vi "Main.vi"(11 "Module Admin":refnum<class "Delacor_lib_QMH_Module Admin.lvclass">) -> ()   [LabVIEW 2025, in "Settings Editor.lvlib"]
doc: "This template is based off of the Queued Message Handler design pattern and the Queued Message Handler project template that ships with LabVIEW.\n\nThe main difference is that the queue is private to this module and communication between modules is performed via Broadcast and Request events.\n\nRequest events are wrapped in public API methods and are handled in the Event Handling Loop (EHL) of this VI. Any module can register for Broadcast events sent by this module. The EHL generates messages based on user interface actions.\n\nThe Message Handling Loop (MHL) processes messages generated by the EHL, or by other messages. The messages are string values, so new messages can be added easily to the Message Cases case structure in the MHL. Each message cluster can also provide an optional value for Message Data, which is a variant that can be converted to whatever message-specific data is required.\n_____\nBased on DQMH Project Template 4.0.0.47.\n_____\nBased on DQMH Dev Tools: Project Template 7.1.0.1503."
uses:
  Settings Editor.lvlib
  <vilib>/Delacor/Delacor QMH/Libraries/Module Admin_class/Delacor_lib_QMH_Module Admin.lvclass
  Test Meta Data.ctl
  Module Data--cluster.ctl
  Settings--cluster.ctl
  Stop Argument--cluster.ctl
  <vilib>/Delacor/Delacor QMH/Libraries/Message Queue_class/Delacor_lib_QMH_Message Queue.lvclass/Delacor_lib_QMH_Message Queue.ctl
  Update Application Settings Argument--cluster.ctl
  Update Application Settings (Reply Payload)--cluster.ctl
  <vilib>/Delacor/Delacor QMH/Libraries/Module Admin_class/Delacor_lib_QMH_Module Admin.lvclass/Delacor_lib_QMH_Module Admin.ctl
  Udate Test Meta Data Argument--cluster.ctl
  Save Test Meta Data (Reply Payload)--cluster.ctl
  <vilib>/Utility/miscctls.llb/LVPointTypeDef.ctl
  <vilib>/Delacor/Delacor QMH/Libraries/Message Queue_class/Delacor_lib_QMH_Enqueue Message (Single).vi
  <vilib>/Delacor/Delacor QMH/Libraries/Module Admin_class/Delacor_lib_QMH_Get External Launch.vi
  <vilib>/Delacor/Delacor QMH/Libraries/Message Queue_class/Delacor_lib_QMH_Message Queue.lvclass
panel:
  in  "Report Save Path":path
  in  "DAQ Settings":T1
  in  "Test Meta Data":T2
  in  "Cancel":bool
  in  "OK":bool
  in  "Log File Base Path":path
  out "error out":errorcluster
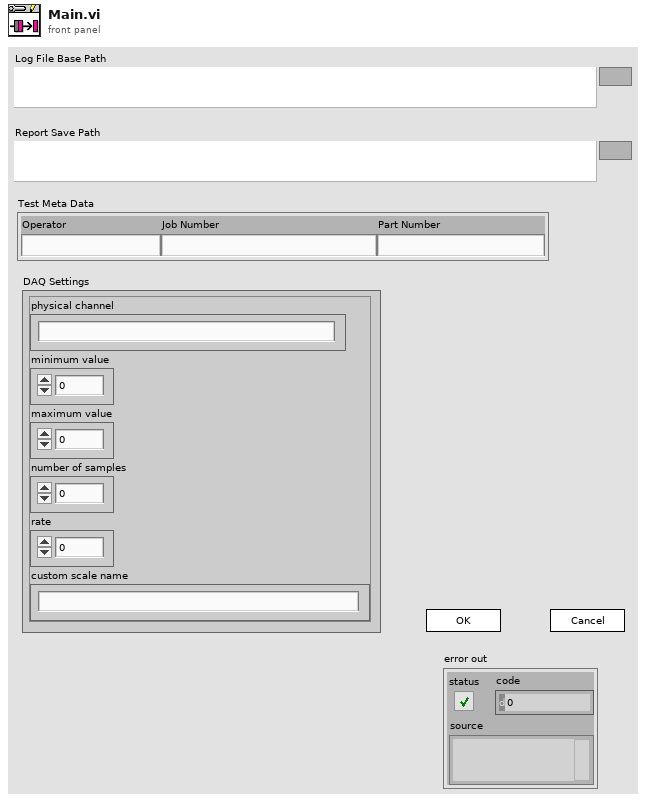
[diagram p1: front panel]
types:
  T1 = cluster{"physical channel":string, "minimum value":dbl, "maximum value":dbl, "number of samples":i32, "rate":dbl, "custom scale name":string}
  T2 = typedef "Settings Editor.lvlib/Test Meta Data.ctl" = cluster{"Operator":string, "Job Number":string, "Part Number":string}
  T3 = typedef "Settings Editor.lvlib/Request Events--cluster.ctl" = cluster{"Stop Module":refnum<user-event>, "Show Panel":refnum<user-event>, "Hide Panel":refnum<user-event>, "Get Module Execution Status":refnum<user-event>, "Show Diagram":refnum<user-event>, "Update Application Settings":refnum<user-event>, "Save Test Meta Data":refnum<user-event>}
  T4 = typedef "Settings Editor.lvlib/Module Data--cluster.ctl" = cluster{"Settings":T5}
  T5 = typedef "Settings Editor.lvlib/Settings--cluster.ctl" = cluster{"Log File Base Path":path, "Meta Data":T2, "DAQ Settings":cluster{"physical channel":string, "minimum value":dbl, "maximum value":dbl, "number of samples":i32, "rate":dbl, "custom scale name":string}, "Report Save Folder":path}
  T6 = enum32{"invalid lock state", "Not Locked", "Locked (No Password)", "Password-protected"}
  T7 = typedef "Settings Editor.lvlib/Stop Argument--cluster.ctl" = cluster{"Origin":string, "Exit via Stop Module Req?":bool, "Wait for Module to stop?":bool}
  T8 = typedef "Settings Editor.lvlib/Update Application Settings Argument--cluster.ctl" = cluster{"Wait Notifier":refnum<notifier>, "wait for reply":bool}
  T9 = typedef "Settings Editor.lvlib/Udate Test Meta Data Argument--cluster.ctl" = cluster{"Test Meta Data":T2, "Wait Notifier":refnum<notifier>, "wait for reply":bool}
  T10 = typedef "LVPointTypeDef.ctl" = cluster{"Horizontal":i16, "Vertical":i16}
  T11 = enum32{"Invalid", "Standard", "Closed", "Hidden", "Minimized", "Maximized"}
  T12 = typedef "Settings Editor.lvlib/Update Application Settings (Reply Payload)--cluster.ctl" = cluster{"Settings":T5, "error":errorcluster}
  T13 = typedef "Settings Editor.lvlib/Save Test Meta Data (Reply Payload)--cluster.ctl" = cluster{"error":errorcluster}
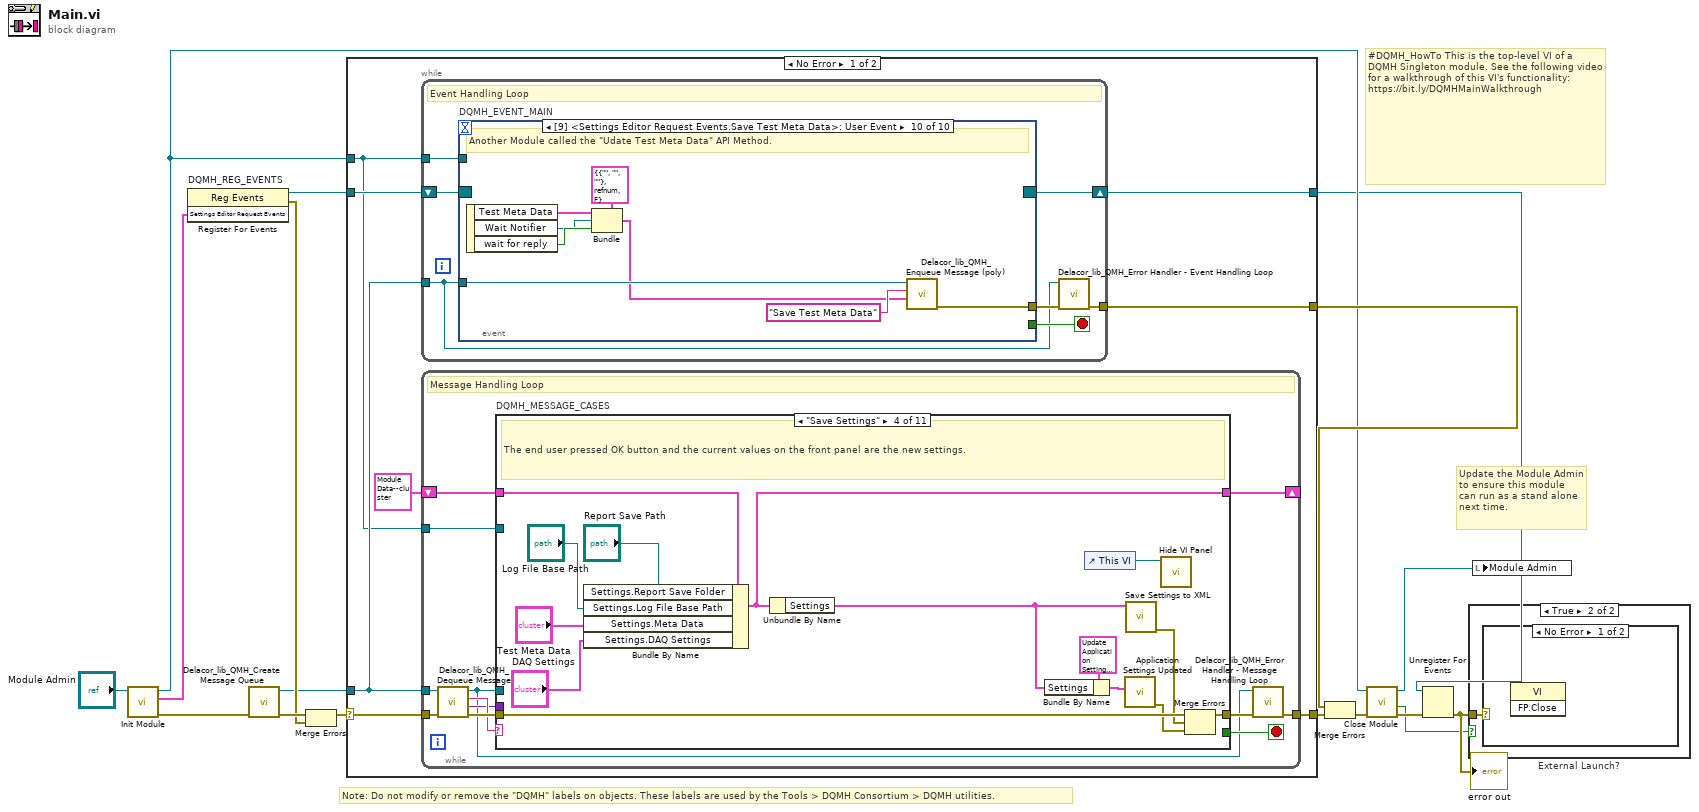
[diagram p0: block diagram]
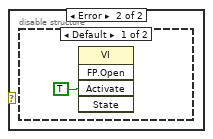
[diagram p3: hidden frame]
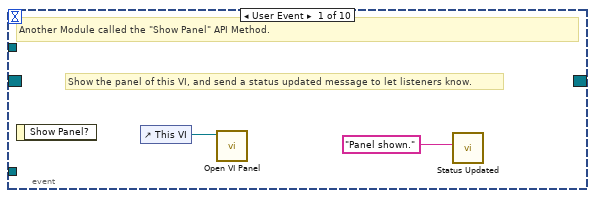
[diagram p5: hidden frame]
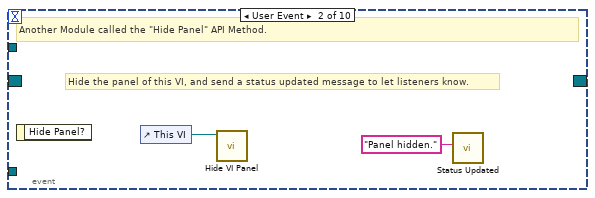
[diagram p6: hidden frame]
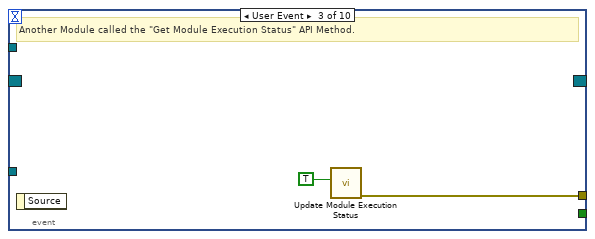
[diagram p7: hidden frame]
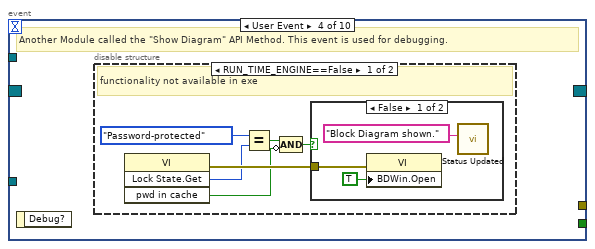
[diagram p8: hidden frame]
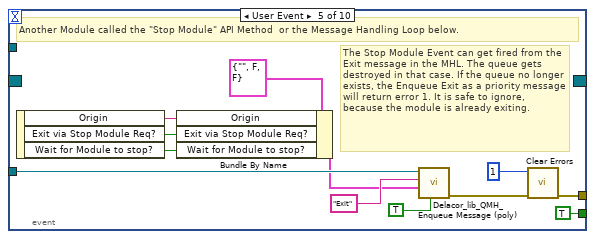
[diagram p11: hidden frame]
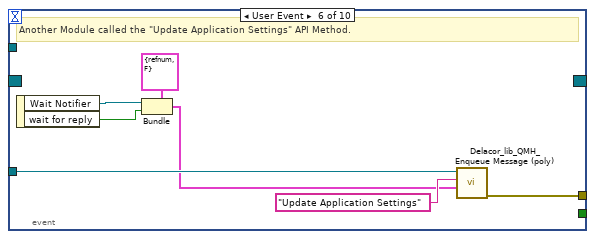
[diagram p12: hidden frame]
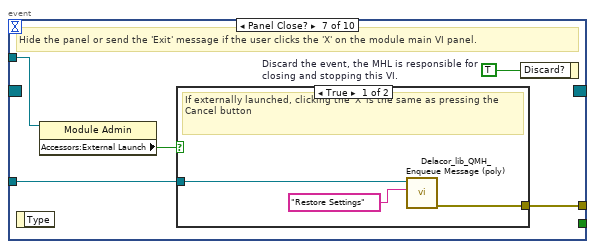
[diagram p13: hidden frame]
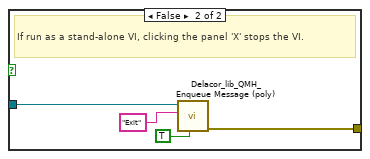
[diagram p14: hidden frame]
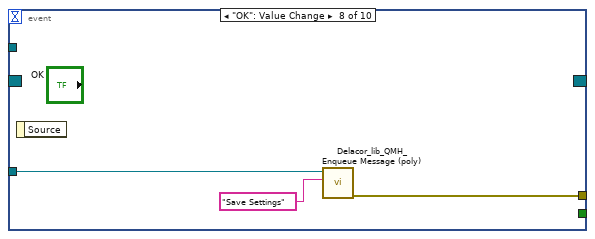
[diagram p15: hidden frame]
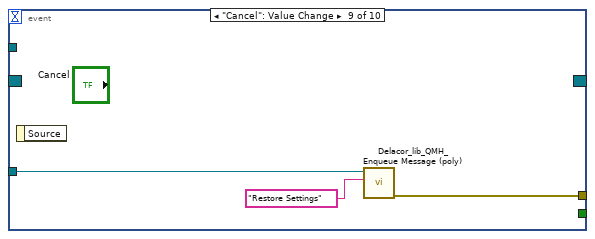
[diagram p16: hidden frame]
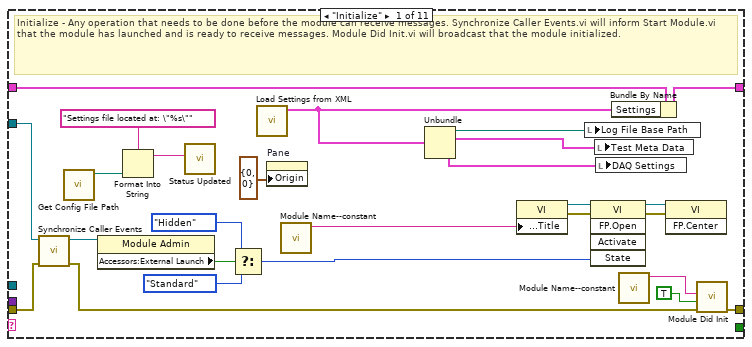
[diagram p17: hidden frame]
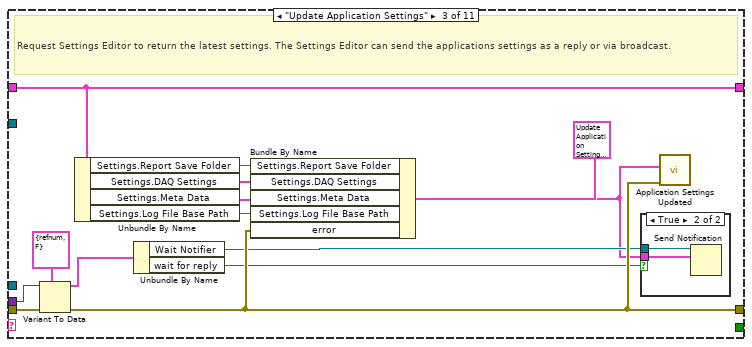
[diagram p19: hidden frame]
diagram:
  # "#DQMH_HowTo This is the top-level VI of a DQMH Singleton module. See the following video for a walkthrough of this VI's functionality: https://bit.ly/DQMHMainWalkthrough"
  # "Note: Do not modify or remove the \"DQMH\" labels on objects. These labels are used by the Tools > DQMH Consortium > DQMH utilities."
  # "Update the Module Admin to ensure this module can run as a stand alone next time."
  n1 = call "Init Module.vi"("Singleton Module Admin in"="Module Admin") -> ("error out"=w16:errorcluster, "Settings Editor Request Events"=w5:T3, "Singleton Module Admin out"=w8:refnum<class "Delacor_lib_QMH_Module Admin.lvclass">)  [unwired: 8 in]
  n2 = register-events "DQMH_REG_EVENTS"(w5) -> (reference out=w6:refnum<event-registration>, error out=w9:errorcluster)  [unwired: 2 in]
  n3 = call <vilib>:"Delacor_lib_QMH_Create Message Queue.vi"("error in"=w16) -> ("error out"=w11:errorcluster, "Message Queue"=w4:refnum<class "Delacor_lib_QMH_Message Queue.lvclass">)  [unwired: 9 in]
  n4 = Merge Errors(w11, w9) -> (w10:errorcluster)
  n5 = case shown="No Error" w10 {
    selector: w10 -> [w23 w244]
    tunnel: [w25 w243] -> w17
    tunnel: [w22 w242] -> w7
    tunnel: w6 -> [w20 w242]
    tunnel: w4 -> [w19 w237]
    tunnel: [w24 _] -> w14
    tunnel: w8 -> [w18 w238]
    frame No Error {
      n6 = while {
        tunnel: w19 -> [w26]
        shift-right: [w29] -> w22
        shift-left: w20 -> [w30]
        tunnel: [w31] -> w24
        tunnel: w18 -> [w27]
        stop <- w28 stop-if-true
        # "Event Handling Loop"
        n7 = event "DQMH_EVENT_MAIN" shown="[9] <Settings Editor Request Events.Save Test Meta Data>: User Event" {
          selector: w30 -> [_ _ _ _ _ _ _ _ _ _]
          dyn-events: [_ _ _ _ _ _ _ _ _ _] -> w29
          timeout: _ -> [_ _ _ _ _ _ _ _ _ _]
          tunnel: [_ _ _ _ TRUE ("Discard?") _ _ _ _ _] -> w28
          tunnel: w26 -> [_ _ _ _ w55 w65 w69 w79 w82 w92]
          tunnel: [_ _ w38 _ w58 w66 w71 w81 w84 w87] -> w32
          tunnel: w27 -> [_ _ _ _ _ _ w68 _ _ _]
          event User Event {
            # "Show the panel of this VI, and send a status updated message to let listeners know."
            # "Another Module called the \"Show Panel\" API Method."
            n8 = event-data() -> ()  [unwired: 1 in, 1 out]
            n9 = control-ref of="This VI"() -> (w34:refnum<vi>)
            n10 = call "Open VI Panel.vi"("VI"=w34) -> ()  [unwired: 10 in, 1 out]
            n11 = call "Status Updated.vi"("Status"="Panel shown." ("format string")) -> ()  [unwired: 10 in, 1 out]
          }
          event User Event {
            # "Hide the panel of this VI, and send a status updated message to let listeners know."
            # "Another Module called the \"Hide Panel\" API Method."
            n12 = event-data() -> ()  [unwired: 1 in, 1 out]
            n13 = control-ref of="This VI"() -> (w36:refnum<vi>)
            n14 = call "Hide VI Panel.vi"("VI"=w36) -> ()  [unwired: 10 in, 1 out]
            n15 = call "Status Updated.vi"("Status"="Panel hidden." ("format string")) -> ()  [unwired: 10 in, 1 out]
          }
          event User Event {
            # "Another Module called the \"Get Module Execution Status\" API Method."
            n16 = event-data() -> ()  [unwired: 1 in, 1 out]
            n17 = call "Update Module Execution Status.vi"("Running?"=TRUE) -> ("error out"=w38:errorcluster)  [unwired: 10 in]
          }
          event User Event {
            # "Another Module called the \"Show Diagram\" API Method. This event is used for debugging."
            n18 = event-data() -> ()  [unwired: 1 in, 1 out]
            n19 = disable-structure shown="RUN_TIME_ENGINE==False" {
              frame condition #0 (active) {
                # "functionality not available in exe"
                n20 = invoke on="Invoke Node" class="VI" method="Lock State.Get"() -> (error out=w44:errorcluster, "Get Lock State"=w43:T6, "pwd in cache"=w40:bool)  [unwired: 4 in, 1 out]
                n21 = Equal?(x=T6."Password-protected", y=w43) -> (x = y?=w41:bool)
                n22 = Compound Arithmetic op=AND(w41, invert w40) -> (w39:bool)
                n23 = case shown="False" w39 {
                  tunnel: w44 -> [w47 _]
                  frame False {
                    n24 = property on="Property Node" class="VI"(error in=w47, "BDWin.Open"=TRUE ("Block Diagram Window:Open")) -> ()  [unwired: 1 in, 2 out]
                    n25 = call "Status Updated.vi"("Status"="Block Diagram shown." ("format string")) -> ()  [unwired: 10 in, 1 out]
                  }
                  frame True {
                    # "Password-protected VI, and the password is not in the cache. Do not show the diagram."
                  }
                }
              }
              frame condition #1 {
              }
            }
          }
          event User Event {
            # "The Stop Module Event can get fired from the Exit message in the MHL. The queue gets destroyed in that case. If the queue no longer exists, the Enqueue Exit as a priority message will return error 1. It is safe to ignore, because the module is already exiting."
            # "Another Module called the \"Stop Module\" API Method  or the Message Handling Loop below."
            n26 = event-data() -> ("Origin"=w48:string, "Exit via Stop Module Req?"=w51:bool, "Wait for Module to stop?"=w50:bool)  [unwired: 1 in]
            n27 = Bundle By Name(cluster=T7 {"Origin"="", "Exit via Stop Module Req?"=FALSE, "Wait for Module to stop?"=FALSE} ("Stop Argument"), "Origin"=w48, "Exit via Stop Module Req?"=w51, "Wait for Module to stop?"=w50) -> (w49:T7)
            n28 = call-poly <vilib>:"Delacor_lib_QMH_Enqueue Message (poly).vi"("Priority Message? (F)"=TRUE, "Message Data"=w49, "Message"="Exit", "Message Queue in"=w55) -> ("error out"=w59:errorcluster)  [unwired: 6 in, 1 out]
            n29 = call <vilib>:"Clear Errors.vi"("error in (no error)"=w59, "specific error code to clear (0: all)"=1) -> ("error out"=w58:errorcluster)  [unwired: 4 in, 1 out]
          }
          event User Event {
            # "Another Module called the \"Update Application Settings\" API Method."
            n30 = event-data() -> ("Wait Notifier"=w61:refnum<notifier>, "wait for reply"=w60:bool)  [unwired: 1 in]
            n31 = Bundle(cluster=T8 {"Wait Notifier"=refnum, "wait for reply"=FALSE} ("Update Application Settings Argument"), "Wait Notifier"=w61, "wait for reply"=w60) -> (w62:T8)
            n32 = call-poly <vilib>:"Delacor_lib_QMH_Enqueue Message (poly).vi"("Message Data"=w62, "Message"="Update Application Settings", "Message Queue in"=w65) -> ("error out"=w66:errorcluster)  [unwired: 7 in, 1 out]
          }
          event Panel Close? {
            w70 = TRUE  # Discard the event, the MHL is responsible for closing and stopping this VI.
            # "Hide the panel or send the 'Exit' message if the user clicks the 'X' on the module main VI panel."
            n33 = event-data() -> ()  [unwired: 1 in, 1 out]
            n34 = property on="Property Node" class="Module Admin"(reference=w68) -> ("Accessors:External Launch"=w67:bool)  [unwired: 1 in, 2 out]
            n35 = case shown="True" w67 {
              tunnel: w69 -> [w72 w77]
              tunnel: [w74 w78] -> w71
              frame True {
                # "If externally launched, clicking the 'X' is the same as pressing the Cancel button"
                n36 = call-poly <vilib>:"Delacor_lib_QMH_Enqueue Message (poly).vi"("Message"="Restore Settings", "Message Queue in"=w72) -> ("error out"=w74:errorcluster)  [unwired: 8 in, 1 out]
              }
              frame False {
                # "If run as a stand-alone VI, clicking the panel 'X' stops the VI."
                n37 = call-poly <vilib>:"Delacor_lib_QMH_Enqueue Message (poly).vi"("Priority Message? (F)"=TRUE, "Message"="Exit", "Message Queue in"=w77) -> ("error out"=w78:errorcluster)  [unwired: 7 in, 1 out]
              }
            }
            n38 = event-data ("Event Filter Node")("Discard?"=w70) -> ()  [unwired: 1 in, 1 out]
          }
          event "OK": Value Change {
            n39 = event-data() -> ()  [unwired: 1 in, 1 out]
            n40 = call-poly <vilib>:"Delacor_lib_QMH_Enqueue Message (poly).vi"("Message"="Save Settings", "Message Queue in"=w79) -> ("error out"=w81:errorcluster)  [unwired: 8 in, 1 out]
          }
          event "Cancel": Value Change {
            n41 = event-data() -> ()  [unwired: 1 in, 1 out]
            n42 = call-poly <vilib>:"Delacor_lib_QMH_Enqueue Message (poly).vi"("Message"="Restore Settings", "Message Queue in"=w82) -> ("error out"=w84:errorcluster)  [unwired: 8 in, 1 out]
          }
          event User Event {
            # "Another Module called the \"Udate Test Meta Data\" API Method."
            n43 = event-data() -> ("Test Meta Data"=w88:T2, "Wait Notifier"=w85:refnum<notifier>, "wait for reply"=w86:bool)  [unwired: 1 in]
            n44 = Bundle(cluster=T9 {"Test Meta Data"={"Operator"="", "Job Number"="", "Part Number"=""}, "Wait Notifier"=refnum, "wait for reply"=FALSE} ("Udate Test Meta Data Argument"), "Test Meta Data"=w88, "Wait Notifier"=w85, "wait for reply"=w86) -> (w89:T9)
            n45 = call-poly <vilib>:"Delacor_lib_QMH_Enqueue Message (poly).vi"("Message Data"=w89, "Message"="Save Test Meta Data", "Message Queue in"=w92) -> ("error out"=w87:errorcluster)  [unwired: 7 in, 1 out]
          }
        }
        n46 = call-dynamic "Delacor_lib_QMH_Error Handler - Event Handling Loop.vi"("error in"=w32, "Message Queue in"=w26) -> ("dup error in"=w31:errorcluster)  [unwired: 8 in, 1 out]
      }
      n47 = while {
        tunnel: w19 -> [w95]
        shift-right: [w99] -> _
        shift-left: T4 {"Settings"={"Log File Base Path"=path "", "Meta Data"={"Operator"="", "Job Number"="", "Part Number"=""}, "DAQ Settings"={"physical channel"="cDAQ9181-1913300Mod1/ai0", "minimum value"=0.0, "maximum value"=94400.0, "number of samples"=10, "rate"=125.0, "custom scale name"="Pressure"}, "Report Save Folder"=path ""}} ("Data Cluster") -> [w100]
        tunnel: w23 -> [w103]
        tunnel: [w101] -> w25
        tunnel: w18 -> [w93]
        stop <- w98 stop-if-true
        # "Message Handling Loop"
        n48 = call-dynamic "Delacor_lib_QMH_Dequeue Message.vi"("error in"=w103, "Message Queue in"=w95) -> ("error out"=w102:errorcluster, "Message Data"=w96:variant, "Message"=w97:string, "Message Queue out"=w94:refnum<class "Delacor_lib_QMH_Message Queue.lvclass">)  [unwired: 6 in]
        n49 = case "DQMH_MESSAGE_CASES" shown="\"Save Settings\"" w97 {
          selector: w97 -> [_ _ _ _ _ _ _ _ _ _ w232]
          tunnel: w94 -> [_ _ _ _ _ _ _ _ w198 w220 _]
          tunnel: w102 -> [w129 w132 w145 w161 w170 w187 w192 w194 w205 w226 w235]
          tunnel: [w127 w132 w146 w162 w170 w178 w191 w194 w201 w221 w236] -> w104
          tunnel: w100 -> [w117 w131 w139 w158 w169 w174 w190 w193 w200 w219 w233]
          tunnel: [w116 w131 w139 w156 w169 w172 w190 w193 w200 w219 w233] -> w99
          tunnel: [_ _ _ _ _ _ _ _ _ w218 _] -> w98
          tunnel: w96 -> [_ _ w144 _ _ w185 _ _ w199 w217 _]
          tunnel: w93 -> [w118 _ _ _ _ _ _ _ w197 w212 _]
          frame "Initialize" {
            # "Initialize - Any operation that needs to be done before the module can receive messages. Synchronize Caller Events.vi will inform Start Module.vi that the module has launched and is ready to receive messages. Module Did Init.vi will broadcast that the module initialized."
            n50 = call "Synchronize Caller Events.vi"("error in"=w129, "Singleton Module Admin in"=w118) -> ("error out"=w128:errorcluster, "Singleton Module Admin out"=w113:refnum<class "Delacor_lib_QMH_Module Admin.lvclass">)  [unwired: 8 in]
            n51 = call "Get Config File Path.vi"() -> ("XML File Path"=w111:path)  [unwired: 10 in, 1 out]
            n52 = property on="Property Node" class="Module Admin"(reference=w113) -> ("Accessors:External Launch"=w122:bool)  [unwired: 1 in, 2 out]
            n53 = Format Into String(format string="Settings file located at: \"%s\"", w111) -> (resulting string=w110:string)  [unwired: 2 in, 1 out]
            n54 = call "Status Updated.vi"("Status"=w110) -> ()  [unwired: 10 in, 1 out]
            n55 = Select(t=T11."Hidden" ("State"), s=w122, f=T11."Standard" ("State")) -> (s? t:f=w119:T11)
            n56 = call "Load Settings from XML.vi"() -> ("Settings out"=w107:T5)  [unwired: 10 in, 1 out]
            n57 = property on="Pane" class="Pane"("Origin"=T10 {"Horizontal"=0, "Vertical"=0}) -> ()  [unwired: 2 in, 2 out]
            n58 = call "Module Name--constant.vi"() -> ("Module Name"=w125:string)  [unwired: 11 in]
            n59 = Unbundle(w107) -> ("Log File Base Path"=w108:path, "Meta Data"=w106:T2, "DAQ Settings"=w105:T1)  [unwired: 1 out]
            n60 = property on="Property Node" class="VI"("Front Panel.Title"=w125) -> (reference out=w124:refnum<vi>, error out=w126:errorcluster)  [unwired: 2 in]
            n61 = local write "Log File Base Path"(w108) -> ()
            n62 = invoke on="Invoke Node" class="VI" method="FP.Open"(reference=w124, error in=w126, "State"=w119) -> (reference out=w123:refnum<vi>, error out=w130:errorcluster)  [unwired: 2 in, 3 out]
            n63 = local write "Test Meta Data"(w106) -> ()
            n64 = local write "DAQ Settings"(w105) -> ()
            n65 = Bundle By Name(cluster=w117, "Settings"=w107) -> (w116:T4)
            n66 = call "Module Name--constant.vi"() -> ("Module Name"=w114:string)  [unwired: 11 in]
            n67 = invoke on="Invoke Node" class="VI" method="FP.Center"(reference=w123, error in=w130) -> ()  [unwired: 1 in, 3 out]
            n68 = call "Module Did Init.vi"("error in"=w128, "Initialized?"=TRUE, "Origin"=w114) -> ("error out"=w127:errorcluster)  [unwired: 8 in]
          }
          frame "---Module Specific---" {
            # "Separator -- The following cases handle messages specific to this Module."
          }
          frame "Update Application Settings" {
            # "Request Settings Editor to return the latest settings. The Settings Editor can send the applications settings as a reply or via broadcast."
            n69 = Variant To Data(error in=w145, type=T8 {"Wait Notifier"=refnum, "wait for reply"=FALSE} ("Update Application Settings Argument"), Variant=w144) -> (data=w142:T8, error out=w146:errorcluster)
            n70 = Unbundle By Name(w139) -> ("Settings.Report Save Folder"=w133:path, "Settings.DAQ Settings"=w134:T1, "Settings.Meta Data"=w135:T2, "Settings.Log File Base Path"=w137:path)
            n71 = Unbundle By Name(w142) -> ("Wait Notifier"=w141:refnum<notifier>, "wait for reply"=w140:bool)
            n72 = Bundle By Name(cluster=T12 {"Settings"={"Log File Base Path"=path "", "Meta Data"={"Operator"="", "Job Number"="", "Part Number"=""}, "DAQ Settings"={"physical channel"="cDAQ9181-1913300Mod1/ai0", "minimum value"=0.0, "maximum value"=94400.0, "number of samples"=10, "rate"=125.0, "custom scale name"="Pressure"}, "Report Save Folder"=path ""}, "error"={"status"=FALSE, "code"=0, "source"=""}} ("Update Application Settings (Reply Payload)"), "Settings.Report Save Folder"=w133, "Settings.DAQ Settings"=w134, "Settings.Meta Data"=w135, "Settings.Log File Base Path"=w137, "error"=w146) -> (w136:T12)
            n73 = case shown="True" w140 {
              tunnel: w141 -> [_ w148]
              tunnel: w136 -> [_ w147]
              frame False {
              }
              frame True {
                n74 = Send Notification(notification=w147, notifier=w148) -> ()  [unwired: 1 in, 2 out]
              }
            }
            n75 = call "Application Settings Updated.vi"("error in"=w146, "Reply Payload"=w136) -> ()  [unwired: 9 in, 1 out]
          }
          frame "Save Settings" {
            # "The end user pressed OK button and the current values on the front panel are the new settings."
            n76 = Bundle By Name(cluster=w158, "Settings.Report Save Folder"="Report Save Path", "Settings.Log File Base Path"="Log File Base Path", "Settings.Meta Data"="Test Meta Data", "Settings.DAQ Settings"="DAQ Settings") -> (w156:T4)
            n77 = Unbundle By Name(w156) -> ("Settings"=w152:T5)
            n78 = Bundle By Name(cluster=T12 {"Settings"={"Log File Base Path"=path "", "Meta Data"={"Operator"="", "Job Number"="", "Part Number"=""}, "DAQ Settings"={"physical channel"="cDAQ9181-1913300Mod1/ai0", "minimum value"=0.0, "maximum value"=94400.0, "number of samples"=10, "rate"=125.0, "custom scale name"="Pressure"}, "Report Save Folder"=path ""}, "error"={"status"=FALSE, "code"=0, "source"=""}} ("Reply Payload"), "Settings"=w152) -> (w153:T12)
            n79 = control-ref of="This VI"() -> (w157:refnum<vi>)
            n80 = call "Application Settings Updated.vi"("Reply Payload"=w153) -> ("error out"=w159:errorcluster)  [unwired: 10 in]
            n81 = call "Save Settings to XML.vi"("Settings"=w152) -> ("error out"=w160:errorcluster)  [unwired: 10 in]
            n82 = call "Hide VI Panel.vi"("VI"=w157) -> ()  [unwired: 10 in, 1 out]
            n83 = Merge Errors(w161, w160, w159) -> (w162:errorcluster)
          }
          frame "Restore Settings" {
            # "The end user pressed Cancel button, need to restore the current stored values for the controls on the front panel. No need to broadcast that the settings changed."
            n84 = Unbundle By Name(w169) -> ("Settings.DAQ Settings"=w164:T1, "Settings.Meta Data"=w168:T2, "Settings.Log File Base Path"=w167:path, "Settings.Report Save Folder"=w163:path)
            n85 = control-ref of="This VI"() -> (w166:refnum<vi>)
            n86 = call "Hide VI Panel.vi"("VI"=w166) -> ()  [unwired: 10 in, 1 out]
            n87 = local write "DAQ Settings"(w164) -> ()
            n88 = local write "Test Meta Data"(w168) -> ()
            n89 = local write "Log File Base Path"(w167) -> ()
            n90 = local write "Report Save Path"(w163) -> ()
            n91 = call "Status Updated.vi"("Status"="Panel hidden." ("format string")) -> ()  [unwired: 10 in, 1 out]
          }
          frame "Save Test Meta Data" {
            n92 = Variant To Data(error in=w187, type=T9 {"Test Meta Data"={"Operator"="", "Job Number"="", "Part Number"=""}, "Wait Notifier"=refnum, "wait for reply"=FALSE} ("Udate Test Meta Data Argument"), Variant=w185) -> (data=w183:T9, error out=w186:errorcluster)
            n93 = Unbundle By Name(w183) -> ("Test Meta Data"=w175:T2, "Wait Notifier"=w182:refnum<notifier>, "wait for reply"=w181:bool)
            n94 = local write "Test Meta Data"(w175) -> ()
            n95 = Bundle By Name(cluster=w174, "Settings.Meta Data"=w175) -> (w172:T4)
            n96 = Unbundle By Name(w172) -> ("Settings"=w173:T5)
            n97 = Bundle By Name(cluster=T12 {"Settings"={"Log File Base Path"=path "", "Meta Data"={"Operator"="", "Job Number"="", "Part Number"=""}, "DAQ Settings"={"physical channel"="cDAQ9181-1913300Mod1/ai0", "minimum value"=0.0, "maximum value"=94400.0, "number of samples"=10, "rate"=125.0, "custom scale name"="Pressure"}, "Report Save Folder"=path ""}, "error"={"status"=FALSE, "code"=0, "source"=""}} ("Reply Payload"), "Settings"=w173) -> (w177:T12)
            n98 = call "Save Settings to XML.vi"("Settings"=w173) -> ("error out"=w171:errorcluster)  [unwired: 10 in]
            n99 = call "Application Settings Updated.vi"("Reply Payload"=w177) -> ()  [unwired: 10 in, 1 out]
            n100 = Bundle By Name(cluster=T13 {"error"={"status"=FALSE, "code"=0, "source"=""}} ("Save Test Meta Data (Reply Payload)"), "error"=w171) -> (w180:T13)
            n101 = Merge Errors(w186, w171) -> (w178:errorcluster)
            n102 = case "DQMH_FIRE_NOTIFIER" shown="True" w181 {
              tunnel: w182 -> [_ w189]
              tunnel: w180 -> [_ w188]
              frame False {
              }
              frame True {
                n103 = Send Notification(notification=w188, notifier=w189) -> ()  [unwired: 1 in, 2 out]
              }
            }
          }
          frame "---Copy This Frame---" {
            # "Duplicate this frame when creating new messages.  Change this comment in the duplicated frame to describe this message."
            n104 = Merge Errors(w192) -> (w191:errorcluster)
          }
          frame "---Exit and Error Handling---" {
            # "Separator - The following cases handle errors and exit messages."
          }
          frame "Error" {
            # "Error - Check the error message data and respond accordingly. This message is sent by the \"Error Handler\" VIs at the end of each loop in this application."
            n105 = property on="Property Node" class="Module Admin"(reference=w197) -> ("Accessors:External Launch"=w196:bool)  [unwired: 1 in, 2 out]
            n106 = Variant To Data(error in=w205, type=errorcluster {"status"=FALSE, "code"=0, "source"=""} ("error constant"), Variant=w199) -> (data=w195:errorcluster, error out=w203:errorcluster)
            n107 = local write "error out"(w195) -> ()
            n108 = call "Error Reported.vi"("Error"=w195) -> ()  [unwired: 10 in, 1 out]
            n109 = case shown="False" w196 {
              tunnel: [w210 _] -> w202
              tunnel: w198 -> [w208 _]
              tunnel: w195 -> [w209 _]
              frame False {
                n110 = disable-structure shown="Default" {
                  disable-tunnel: w209 -> [w211 _]
                  frame condition #0 (active) {
                    # "If the module is running standalone, then pop up an error dialog and call the \"Exit\" message."
                    n111 = call <vilib>:"Simple Error Handler.vi"("error in (no error)"=w211) -> ()  [unwired: 4 in, 5 out]
                  }
                  frame condition #1 {
                    # "To prevent the Simple Error Handler VI from being loaded (e.g. when deploying to a Real-Time target), add the Conditional Disable Symbol \"DQMH_Disable_SEH\" to your project and set it to TRUE."
                  }
                }
                n112 = call-poly <vilib>:"Delacor_lib_QMH_Enqueue Message (poly).vi"("Priority Message? (F)"=TRUE, "Message"="Exit", "Message Queue in"=w208) -> ("error out"=w210:errorcluster)  [unwired: 7 in, 1 out]
              }
              frame True {
                # "If the module was launched externally, calling the Error Reported broadcast VI is the only action performed by the \"Error\" message. The module's caller can then process the error appropriately."
              }
            }
            n113 = Merge Errors(w203, w202) -> (w201:errorcluster)
          }
          frame "Exit" {
            w218 = TRUE  # Stop the VI
            # "Release the message queue reference"
            # "Exit - Exit the application."
            n114 = Variant To Data(error in=w226, type=T7 {"Origin"="", "Exit via Stop Module Req?"=FALSE, "Wait for Module to stop?"=FALSE} ("Stop Argument"), Variant=w217) -> (data=w214:T7, error out=w223:errorcluster)
            n115 = call <vilib>:"Clear Errors.vi"("error in (no error)"=w223, "specific error code to clear (0: all)"=91 ("91: not all Exit messages will have an argument")) -> ("error out"=w225:errorcluster)  [unwired: 4 in, 1 out]
            n116 = control-ref of="This VI"() -> (w213:refnum<vi>)
            n117 = call-dynamic "Delacor_lib_QMH_Release Message Queue.vi"("error in"=w225, "Message Queue"=w220) -> ("error out"=w224:errorcluster)  [unwired: 9 in]
            n118 = call "Handle Exit.vi"("Stop Argument"=w214, "Admin in"=w212, "VI reference"=w213) -> ("error out"=w222:errorcluster)  [unwired: 7 in, 1 out]
            n119 = Merge Errors(w224, w222) -> (w221:errorcluster)
            n120 = call "Error Reported.vi"("Error"=w221) -> ()  [unwired: 10 in, 1 out]
          }
          frame Default {
            # "'Default' case only runs if there is a message that isn't defined in any of the other cases.  Output a programming error."
            n121 = call "Module Name--constant.vi"() -> ("Module Name"=w231:string)  [unwired: 11 in]
            n122 = Format Into String(format string="The invalid message string \"%s\" was received in the Message Handling Loop for module \"%s\".", w232, w231) -> (resulting string=w229:string)  [unwired: 2 in, 1 out]
            n123 = call <vilib>:"Error Cluster From Error Code.vi"("show call chain? (False)"=TRUE, "error message (\"\")"=w229, "error code (0)"=1) -> ("error out"=w234:errorcluster)  [unwired: 6 in]
            n124 = Merge Errors(w235, w234) -> (w236:errorcluster)
          }
        }
        n125 = call-dynamic "Delacor_lib_QMH_Error Handler - Message Handling Loop.vi"("error in"=w104, "Message Queue in"=w94) -> ("dup error in"=w101:errorcluster)  [unwired: 8 in, 1 out]
      }
    }
    frame Error {
      # "Synchronize Caller Events.vi will inform Start Module.vi that the module has launched and will let the code calling Start Module.vi register for broadcasts and would permit the caller receive the broadcast that an error occurred at launch time."
      n126 = call "Synchronize Caller Events.vi"("Singleton Module Admin in"=w238) -> ("error out"=w245:errorcluster)  [unwired: 9 in, 1 out]
      n127 = call-dynamic "Delacor_lib_QMH_Release Message Queue.vi"("error in"=w244, "Message Queue"=w237) -> ("error out"=w243:errorcluster)  [unwired: 9 in]
      n128 = call "Module Name--constant.vi"() -> ("Module Name"=w241:string)  [unwired: 11 in]
      n129 = Format Into String(format string="An error occurred during initialization. %s is no longer running.", w241) -> (resulting string=w239:string)  [unwired: 2 in, 1 out]
      n130 = Merge Errors(w243, w245) -> (w246:errorcluster)
      n131 = call "Error Reported.vi"("Additional Information"=w239, "Error"=w246) -> ()  [unwired: 9 in, 1 out]
    }
  }
  n132 = Merge Errors(w14, w17) -> (w13:errorcluster)
  n133 = call "Close Module.vi"("error in"=w13, "Module Admin in"=w8) -> ("error out"=w15:errorcluster, "External Launch"=w1:bool, "Module Admin out"=w2:refnum<class "Delacor_lib_QMH_Module Admin.lvclass">)  [unwired: 7 in]
  n134 = Unregister For Events(event registration refnum=w7, error in=w15) -> (error out=w12:errorcluster)
  "error out" <- w12
  n135 = case "External Launch?" shown="True" w1 {
    tunnel: w12 -> [_ w247]
    frame False {
    }
    frame True {
      n136 = case shown="No Error" w247 {
        frame No Error {
          n137 = invoke on="Invoke Node" class="VI" method="FP.Close"() -> ()  [unwired: 3 in, 3 out]
        }
        frame Error {
          n138 = disable-structure shown="Default" {
            frame condition #0 (active) {
              n139 = invoke class="VI" method="FP.Open"("Activate"=TRUE ("Activate?")) -> ()  [unwired: 4 in, 5 out]
            }
            frame condition #1 {
              # "Don't show panel on error if running inside a built EXE."
            }
          }
        }
      }
    }
  }
  n140 = local write "Module Admin"(w2) -> ()
